vi "Part 1.vi"(11 "Input":string) -> (3 "Output":i64)   [LabVIEW 2021]
uses:
  <userlib>/_OpenG.lib/string/string.llb/Convert EOLs (String)__ogtk.vi
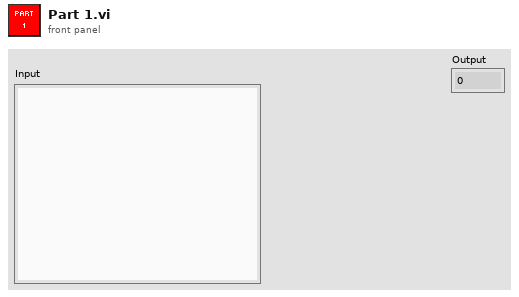
[diagram p1: front panel]
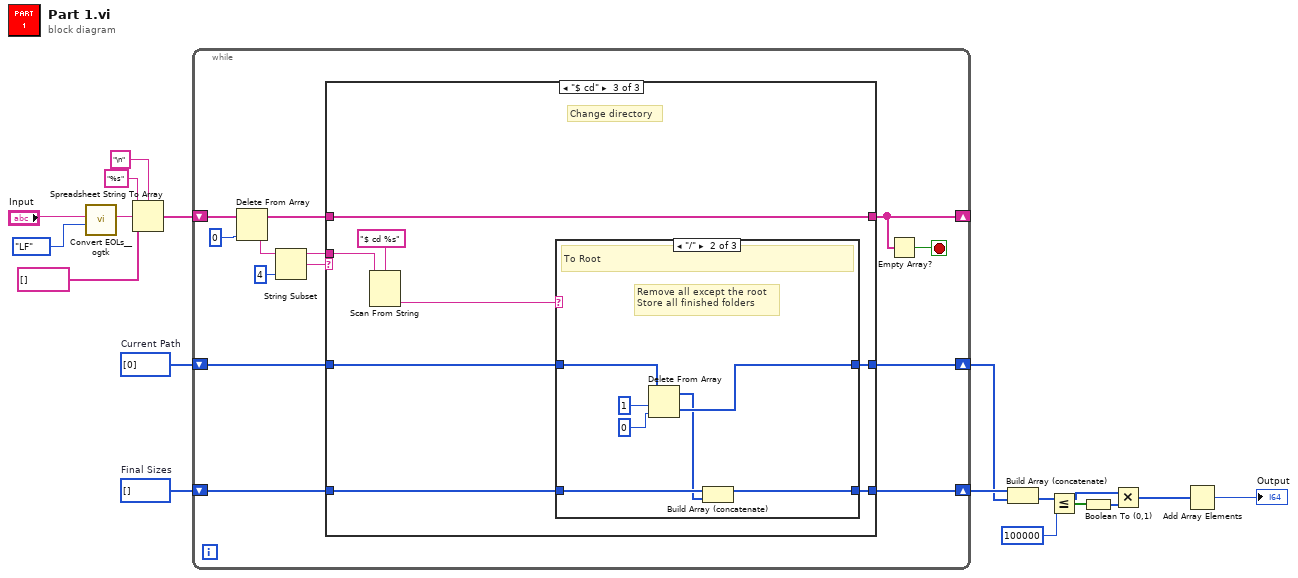
[diagram p0: block diagram]
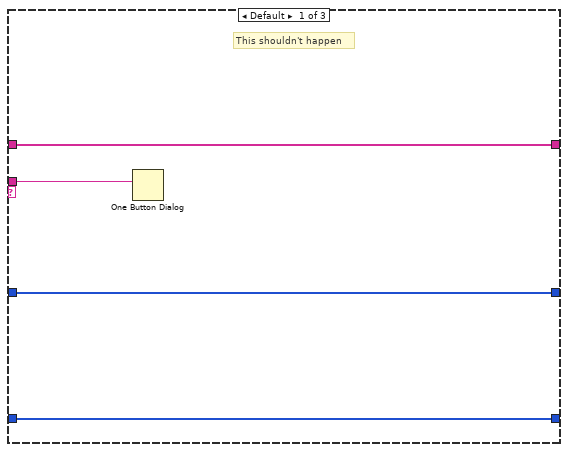
[diagram p2: hidden frame]
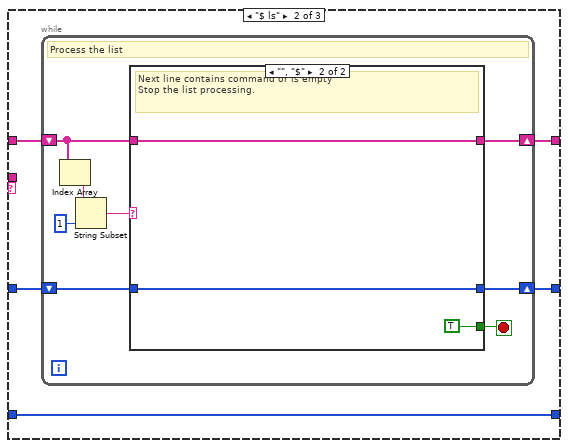
[diagram p3: hidden frame]
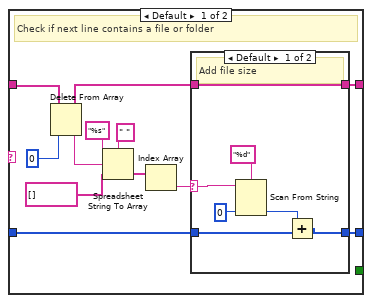
[diagram p4: hidden frame]
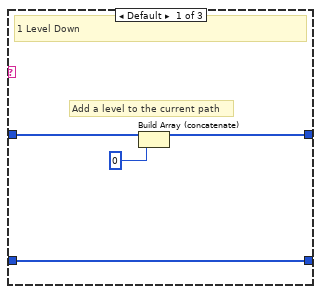
[diagram p6: hidden frame]
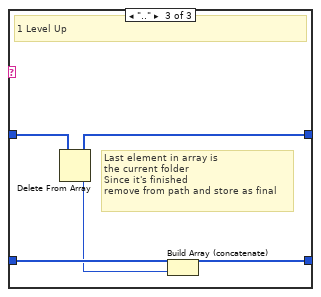
[diagram p7: hidden frame]
diagram:
  w9 = i64[] []  # Final Sizes
  w10 = i64[] [0]  # Current Path
  n1 = call-poly <userlib>:"Convert EOLs__ogtk.vi"("Convert to:"=enum16{"CR", "LF", "CRLF"}."LF", "String in"="Input") -> ("String out"=w16:string)  [unwired: 9 in]
  n2 = Spreadsheet String To Array(delimiter (Tab)="\n", format string="%s", spreadsheet string=w16, array type (2D Dbl)=string[] []) -> (array=w11:string[])
  n3 = while {
    shift-right: [w24] -> _
    shift-left: w11 -> [w29]
    shift-right: [w20] -> w7
    shift-left: w10 -> [w22]
    shift-right: [w18] -> w8
    shift-left: w9 -> [w19]
    stop <- w23 stop-if-true
    n4 = Delete From Array(array=w29, index=0) -> (deleted portion=w21:string, array with subset deleted=w25:string[])  [unwired: 1 in]
    n5 = String Subset(string=w21, length (rest)=4 ("length (rest)")) -> (substring=w26:string)  [unwired: 1 in]
    n6 = case shown="\"$ cd\"" w26 {
      tunnel: w25 -> [w33 w37 w78]
      tunnel: [w33 w36 w78] -> w24
      tunnel: w22 -> [w32 w35 w74]
      tunnel: w21 -> [w30 _ w77]
      tunnel: [w32 w34 w73] -> w20
      tunnel: w19 -> [w31 w38 w72]
      tunnel: [w31 w38 w71] -> w18
      frame Default {
        # "This shouldn't happen"
        n7 = One Button Dialog(message=w30) -> ()  [unwired: 1 in, 1 out]
      }
      frame "$ ls" {
        n8 = while {
          shift-right: [w42] -> w36
          shift-left: w37 -> [w43]
          shift-right: [w40] -> w34
          shift-left: w35 -> [w41]
          stop <- w39 stop-if-true
          # "Process the list"
          n9 = Index Array(array=w43) -> (element=w46:string)  [unwired: 1 in]
          n10 = String Subset(string=w46, length (rest)=1 ("length (rest)")) -> (substring=w44:string)  [unwired: 1 in]
          n11 = case shown="\"\", \"$\"" w44 {
            tunnel: w43 -> [w57 w70]
            tunnel: [w50 w70] -> w42
            tunnel: w41 -> [w48 w69]
            tunnel: [w49 w69] -> w40
            tunnel: [_ TRUE] -> w39
            frame Default {
              # "Check if next line contains a file or folder"
              n12 = Delete From Array(array=w57, index=0) -> (deleted portion=w56:string, array with subset deleted=w51:string[])  [unwired: 1 in]
              n13 = Spreadsheet String To Array(delimiter (Tab)=" ", format string="%s", spreadsheet string=w56, array type (2D Dbl)=string[] []) -> (array=w53:string[])
              n14 = Index Array(array=w53) -> (element=w52:string)  [unwired: 1 in]
              n15 = case shown="Default" w52 {
                selector: w52 -> [w65 _]
                tunnel: w51 -> [w61 w67]
                tunnel: [w61 w67] -> w50
                tunnel: [w59 w66] -> w49
                tunnel: w48 -> [w63 w66]
                frame Default {
                  # "Add file size"
                  n16 = Scan From String(format string="%d", input string=w65, default 1=i64 0) -> (output 1=w62:i64)  [unwired: 2 in, 3 out]
                  n17 = Add(x=w62, y=w63) -> (x+y=w59:i64[])
                }
                frame "dir" {
                  # "Folders will be processed\nThis line doesn't change\nthe sizes"
                  # "Ignore folder"
                }
              }
            }
            frame "", "$" {
              # "Next line contains command or is empty\nStop the list processing."
            }
          }
        }
      }
      frame "$ cd" {
        # "Change directory"
        n18 = Scan From String(format string="$ cd %s", input string=w77) -> (output 1=w75:string)  [unwired: 3 in, 3 out]
        n19 = case shown="\"/\"" w75 {
          tunnel: w74 -> [w81 w86 w93]
          tunnel: [w79 w87 w94] -> w73
          tunnel: w72 -> [w82 w85 w92]
          tunnel: [w82 w83 w90] -> w71
          frame Default {
            # "Add a level to the current path"
            # "1 Level Down"
            n20 = Build Array (concatenate)(w81, i64 0) -> (w79:i64[])
          }
          frame "/" {
            # "Remove all except the root\nStore all finished folders"
            # "To Root"
            n21 = Delete From Array(array=w86, length=1, index=0) -> (deleted portion=w87:i64[], array with subset deleted=w84:i64[])
            n22 = Build Array (concatenate)(w85, w84) -> (w83:i64[])
          }
          frame ".." {
            # "Last element in array is\nthe current folder\nSince it's finished\nremove from path and store as final"
            # "1 Level Up"
            n23 = Delete From Array(array=w93) -> (deleted portion=w91:i64, array with subset deleted=w94:i64[])  [unwired: 2 in]
            n24 = Build Array (concatenate)(w92, w91) -> (w90:i64[])
          }
        }
      }
    }
    n25 = Empty Array?(array=w24) -> (empty?=w23:bool)
  }
  n26 = Build Array (concatenate)(w8, w7) -> (w4:i64[])
  n27 = Less Or Equal?(x=w4, y=i64 100000) -> (x <= y?=w5:bool[])
  n28 = Boolean To (0,1)(Boolean=w5) -> (0, 1=w3:i16[])
  n29 = Multiply(x=w4, y=w3) -> (x*y=w2:i64[])
  n30 = Add Array Elements(numeric array=w2) -> (sum=→"Output":i64)
